vi "sensirion data array to logstring (sub-vi).vi"(5 "line ending (none)":string, 6 "float precision (8)":i16=8, 7 "delimeter (comma)":string=",", 8 "error in":errorcluster, 9 "timestamp in relative seconds":dbl format="%_19f", 10 "sensor data array":T1[](array[typedef]) {"temperature" scale=293.15..303.15 scale format="%#_3g"}, 11 "value format (%15s)":string="%15s") -> (0 "error out":errorcluster, 2 "string out":string)   [LabVIEW 2021]
uses:
  controls/sensirion_flow_sensor_data.ctl
  <vilib>/Utility/error.llb/Error Cluster From Error Code.vi
  <vilib>/ErrorRing/Error Ring.xnode
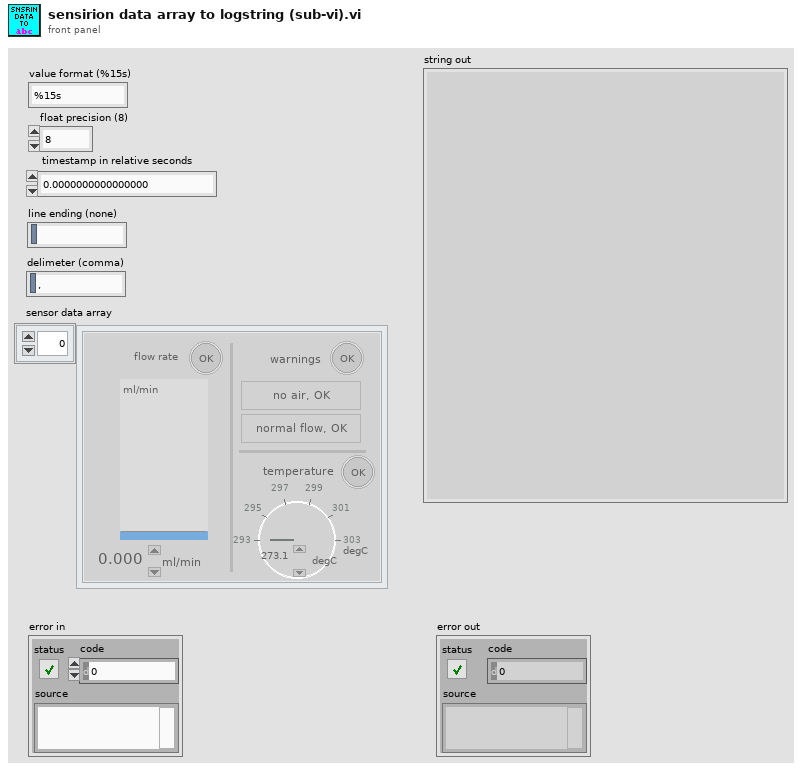
[diagram p1: front panel]
types:
  T1 = typedef "sensirion_flow_sensor_data.ctl" = cluster{"flow rate \n":dbl[unit], "flow val. status":bool, "temperature":dbl[unit], "temp. val status":bool, "air in line?":bool, "high flow?":bool, "flag. val status":bool}
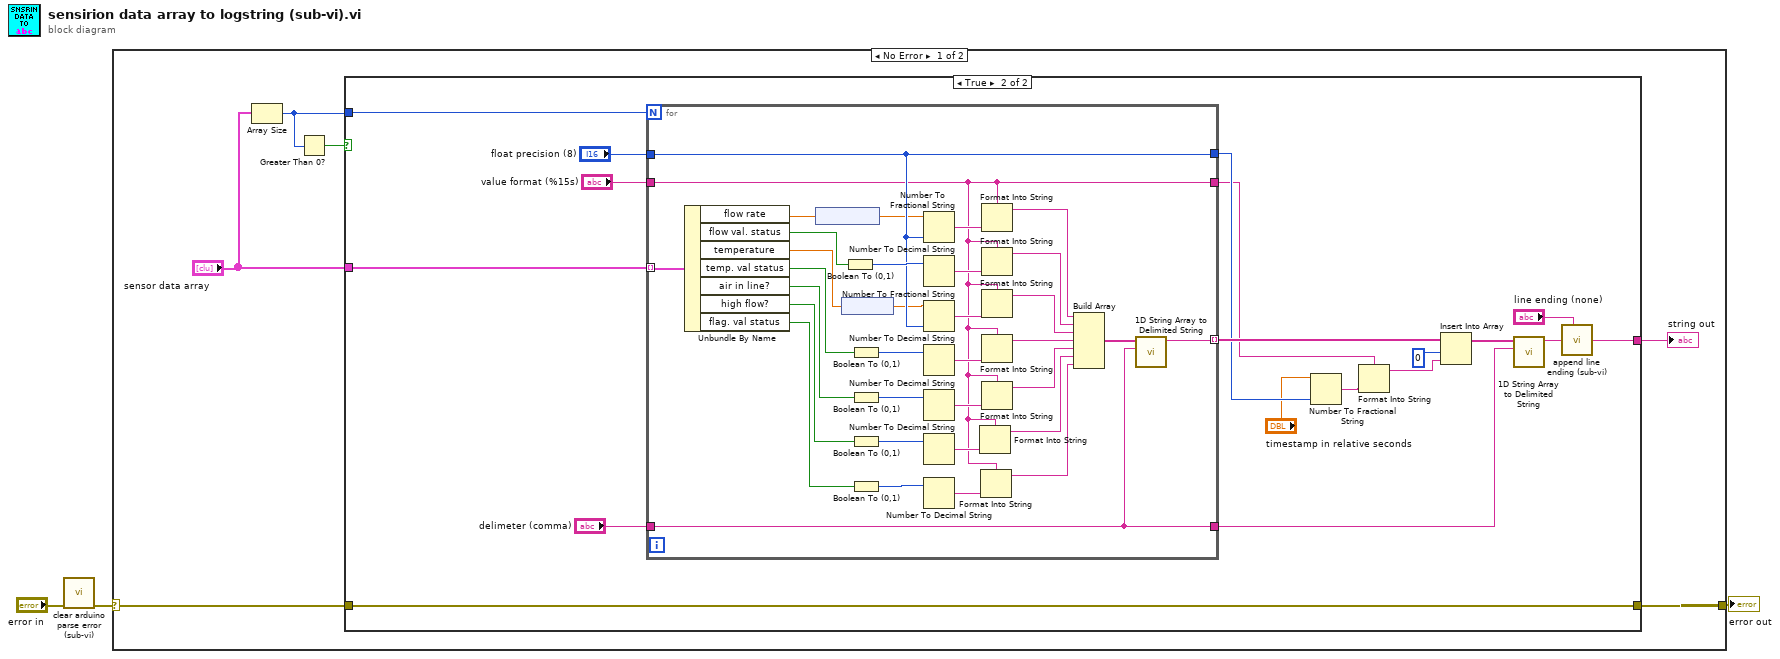
[diagram p0: block diagram]
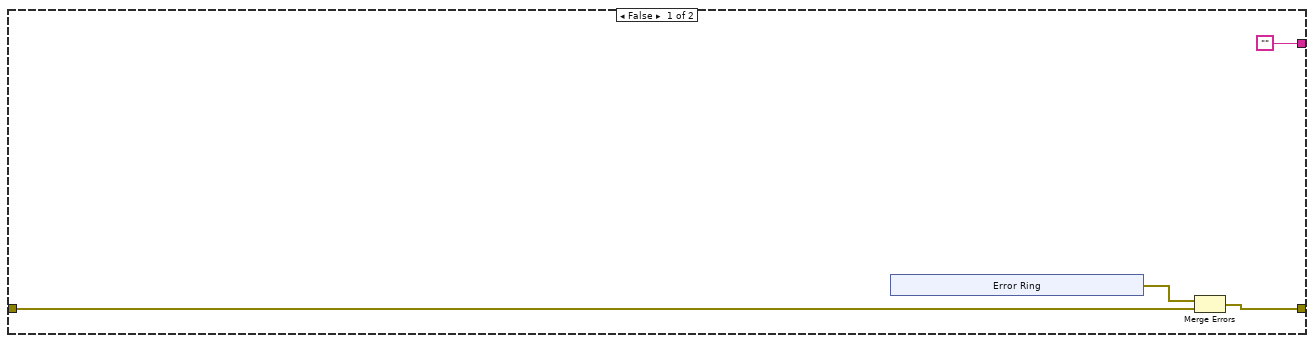
[diagram p2: hidden frame]
diagram:
  n1 = call "clear arduino parse error (sub-vi).vi"("error in"="error in") -> ("error out"=w2:errorcluster)  [unwired: 10 in]
  n2 = case shown="No Error" w2 {
    selector: w2 -> [w5 w70]
    tunnel: [w6 w70] -> w3
    frame No Error {
      n3 = Array Size(array="sensor data array") -> (size(s)=w8:i32)
      n4 = Greater Than 0?(x=w8) -> (x > 0?=w7:bool)
      n5 = case shown="True" w7 {
        tunnel: "sensor data array" -> [_ w35]
        tunnel: w8 -> [_ w34]
        tunnel: [w12 w25] -> w6
        tunnel: w5 -> [w11 w25]
        tunnel: ["" ("string out") w18] -> w4
        frame False {
          n6 = xnode "Error Ring"() -> ("error out"=w13:errorcluster)
          n7 = Merge Errors(w13, w11) -> (w12:errorcluster)
        }
        frame True {
          n8 = for {
            N: w34 -> [_]
            tunnel: w35 -> [w69] mode=indexing
            tunnel: "delimeter (comma)" -> [w55]
            tunnel: [w56] -> w31 mode=indexing
            tunnel: [w55] -> w32
            tunnel: "float precision (8)" -> [w54]
            tunnel: [w54] -> w26
            tunnel: "value format (%15s)" -> [w39]
            tunnel: [w39] -> w20
            n9 = Unbundle By Name(w69) -> ("flow rate"=w68:dbl[unit], "flow val. status"=w67:bool, "temperature"=w37:dbl[unit], "temp. val status"=w66:bool, "air in line?"=w65:bool, "high flow?"=w64:bool, "flag. val status"=w63:bool)
            n10 = node(w68) -> (w38:dbl)
            n11 = node(w37) -> (w36:dbl)
            n12 = Boolean To (0,1)(Boolean=w67) -> (0, 1=w62:i16)
            n13 = Boolean To (0,1)(Boolean=w66) -> (0, 1=w61:i16)
            n14 = Boolean To (0,1)(Boolean=w65) -> (0, 1=w60:i16)
            n15 = Boolean To (0,1)(Boolean=w64) -> (0, 1=w59:i16)
            n16 = Boolean To (0,1)(Boolean=w63) -> (0, 1=w58:i16)
            n17 = Number To Fractional String(number=w38, precision (6)=w54) -> (F-format string=w50:string)  [unwired: 2 in]
            n18 = Number To Decimal String(number=w62) -> (decimal integer string=w51:string)  [unwired: 1 in]
            n19 = Number To Fractional String(number=w36, precision (6)=w54) -> (F-format string=w48:string)  [unwired: 2 in]
            n20 = Number To Decimal String(number=w61) -> (decimal integer string=w46:string)  [unwired: 1 in]
            n21 = Number To Decimal String(number=w60) -> (decimal integer string=w44:string)  [unwired: 1 in]
            n22 = Number To Decimal String(number=w59) -> (decimal integer string=w42:string)  [unwired: 1 in]
            n23 = Number To Decimal String(number=w58) -> (decimal integer string=w40:string)  [unwired: 1 in]
            n24 = Format Into String(format string=w39, w42) -> (resulting string=w43:string)  [unwired: 2 in, 1 out]
            n25 = Format Into String(format string=w39, w40) -> (resulting string=w41:string)  [unwired: 2 in, 1 out]
            n26 = Format Into String(format string=w39, w50) -> (resulting string=w53:string)  [unwired: 2 in, 1 out]
            n27 = Format Into String(format string=w39, w51) -> (resulting string=w52:string)  [unwired: 2 in, 1 out]
            n28 = Format Into String(format string=w39, w48) -> (resulting string=w49:string)  [unwired: 2 in, 1 out]
            n29 = Format Into String(format string=w39, w46) -> (resulting string=w47:string)  [unwired: 2 in, 1 out]
            n30 = Format Into String(format string=w39, w44) -> (resulting string=w45:string)  [unwired: 2 in, 1 out]
            n31 = Build Array(w53, w52, w49, w47, w45, w43, w41) -> (w57:string[])
            n32 = call <vilib>:"1D String Array to Delimited String.vi"("delimiter"=w55, "string array"=w57) -> ("delimited string"=w56:string)  [unwired: 9 in]
          }
          n33 = Number To Fractional String(number="timestamp in relative seconds", precision (6)=w26) -> (F-format string=w19:string)  [unwired: 2 in]
          n34 = Format Into String(format string=w20, w19) -> (resulting string=w21:string)  [unwired: 2 in, 1 out]
          n35 = Insert Into Array(array=w31, index=0, new element=w21) -> (w29:string[])
          n36 = call <vilib>:"1D String Array to Delimited String.vi"("delimiter"=w32, "string array"=w29) -> ("delimited string"=w28:string)  [unwired: 9 in]
          n37 = call "append line ending (sub-vi).vi"("line ending (\\r\\n)"="line ending (none)", "string in"=w28) -> ("string out"=w18:string)  [unwired: 7 in]
        }
      }
      "string out" <- w4
    }
    frame Error {
    }
  }
  "error out" <- w3
